vi "HEWH Get Statistics.vi"(4 "Use Emerson 5700?":bool, 6 "Emerson Flow Meter Data Output":T1, 8 "Error In":errorcluster, 10 "Elapsed Time (sec)":dbl, 11 "Core HEWH Data in":T2 {"Test Patten Setup"."PRAT/RLT Sequence"."Time" format="%<%H:%M:%S>t"; "Test Patten Setup"."Total Gallons Schedule" format="%.2f"}) -> (0 "Error Out":errorcluster, 1 "Mean,SD,Var,Max,Min Array":string[][](array[string]), 3 "Draw Stats Out":dbl[][](array[numeric]))   [LabVIEW 2016]
uses:
  Type Definitions/HEWH Output Information.ctl
  Type Definitions/HEWH Draw Pattern Setup.ctl
  Type Definitions/PRAT Test.ctl
  Utility/Save File/File Setup (Public)/Type Definition/Save File HEWH Heating Control Mode.ctl
  Draw Water Specific/Type Definitions/Terminate Draw Conditions.ctl
  Type Definitions/HEWH Start Conditions.ctl
  Draw Water Specific/Type Definitions/Check Special Condtions.ctl
  Draw Water Specific/Type Definitions/HEWH Special Condition Check.ctl
  Type Definitions/HEWH Draw Flag ENUM.ctl
  Type Definitions/HEWH Specific DAQ.ctl
  Type Definitions/HEWH Power Data.ctl
  Type Definitions/HEWH Power Elements.ctl
  Utility/Type Definitions/UTILITY Power Analyzer.ctl
  Type Definitions/HEWH Calc and Calibration.ctl
  Utility/Save File/File Setup (Public)/Type Definition/Save File DOE LabView Program.ctl
  Custom Instrument Control/MW100/Type Definitions/Station ID Selector.ctl
  Drivers/Emerson 5700 Transmitter/Type Definitions/Emerson 5700 Data.ctl
  Utility/Save File/File Setup.lvlib
panel:
  # "Draw Pattern Setup (24 Hour)"
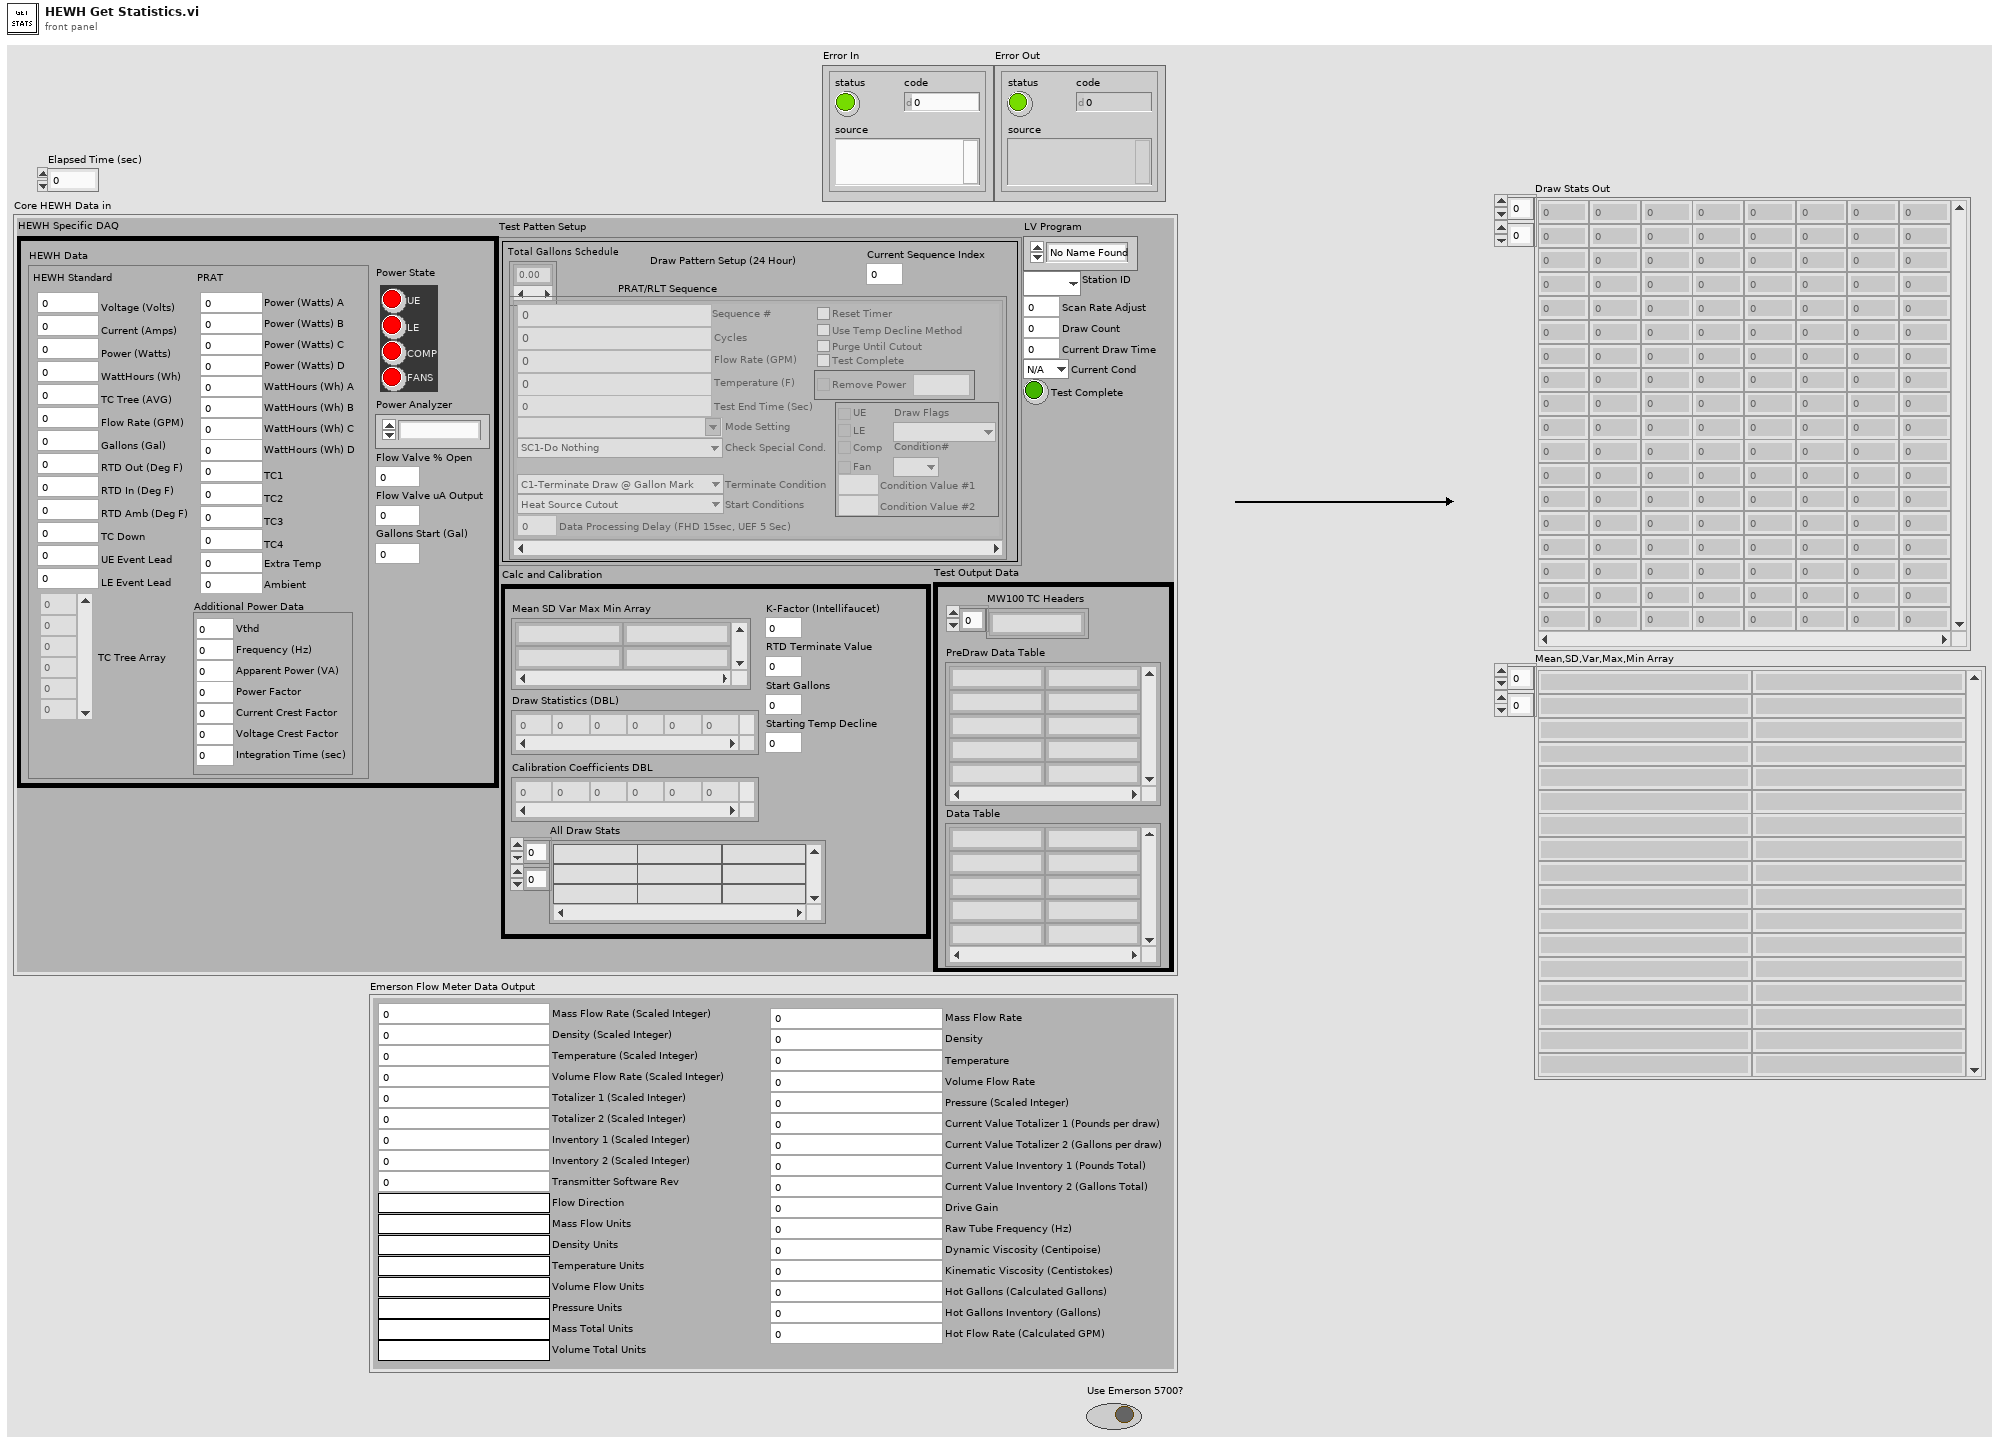
[diagram p1: front panel]
types:
  T1 = typedef "Emerson 5700 Data.ctl" = cluster{"Mass Flow Rate (Scaled Integer)":u16, "Density (Scaled Integer)":u16, "Temperature (Scaled Integer)":u16, "Volume Flow Rate (Scaled Integer)":u16, "Totalizer 1 (Scaled Integer)":u16, "Totalizer 2 (Scaled Integer)":u16, "Transmitter Software Rev":u16, "Flow Direction":string, "Mass Flow Units":string, "Density Units":string, "Temperature Units":string, "Volume Flow Units":string, "Pressure Units":string, "Mass Total Units":string, "Volume Total Units":string, "Inventory 1 (Scaled Integer)":u16, "Inventory 2 (Scaled Integer)":u16, "Mass Flow Rate":dbl, "Density":dbl, "Temperature":dbl, "Volume Flow Rate":dbl, "Pressure (Scaled Integer)":u16, "Current Value Totalizer 1 (Pounds per draw)":dbl, "Current Value Totalizer 2 (Gallons per draw)":dbl, "Current Value Inventory 1 (Pounds Total)":dbl, "Current Value Inventory 2 (Gallons Total)":dbl, "Drive Gain":dbl, "Raw Tube Frequency (Hz)":dbl, "Dynamic Viscosity (Centipoise)":dbl, "Kinematic Viscosity (Centistokes)":dbl, "Hot Gallons (Calculated Gallons)":dbl, "Hot Flow Rate (Calculated GPM)":dbl, "Hot Gallons Inventory (Gallons)":dbl}
  T2 = typedef "HEWH Output Information.ctl" = cluster{"Scan Rate Adjust":dbl, "Draw Count":i32, "Test Patten Setup":T3, "HEWH Specific DAQ":T11, "Test Output Data":cluster{"PreDraw Data Table":string[][], "Data Table":string[][], "MW100 TC Headers":string[]}, "Calc and Calibration":T15, "Current Draw Time":dbl, "LV Program":T16, "Station ID":T17, "Current Cond":T9, "Test Complete":bool}
  T3 = typedef "HEWH Draw Pattern Setup.ctl" = cluster{"Total Gallons Schedule":dbl[], "PRAT/RLT Sequence":T4[], "Current Sequence Index":i32}
  T4 = typedef "PRAT Test.ctl" = cluster{"Sequence #":dbl, "Cycles":i32, "Mode Setting":T5, "Flow Rate (GPM)":dbl, "Temperature (F)":dbl, "Reset Timer":bool, "Use Temp Decline Method":bool, "Terminate Condition":T6, "Condition Value #1":dbl, "UE":bool, "LE":bool, "Comp":bool, "Fan":bool, "Test End Time (Sec)":dbl, "Purge Until Cutout":bool, "Start Conditions":T7, "Condition Value #2":dbl, "Remove Power":bool, "Time":dbl, "Check Special Cond.":T8, "Condition#":T9, "Draw Flags":T10, "Data Processing Delay (FHD 15sec, UEF 5 Sec)":dbl, "Test Complete":bool}
  T5 = typedef "File Setup.lvlib/Save File HEWH Heating Control Mode.ctl" = string
  T6 = typedef "Terminate Draw Conditions.ctl" = enum16{"C1-Terminate Draw @ Gallon Mark", "C2-Special Last Draw (HU Test)", "C3-RTD Out <=", "C4-Mean Tank Temp <=", "C5-Decrease RTD Out (Deg F)", "C6-Time (Seconds)", "C7-Until Any Heat Source", "C8-Specific Heat Source", "C9-Do Nothing"}
  T7 = typedef "HEWH Start Conditions.ctl" = enum16{"Heat Source Cutout", "At Time (Seconds)", "Every X (Seconds)", "T2 >= X° Below Setpoint", "Seconds From Complete", "Wait for LE & Comp Cutout", "Wait for Comp Cutout", "Wait for LE Cutout", "Wait for UE Cutout"}
  T8 = typedef "Check Special Condtions.ctl" = enum16{"SC1-Do Nothing", "SC2-Check Heat Source (On-C2/Off-C1)", "SC3-Check Skip Condition", "SC4-Check Heat Source ON/Fail"}
  T9 = typedef "HEWH Special Condition Check.ctl" = enum16{"N/A", "C1", "C2", "Reset/Fail", "Skip Draw Sequence"}
  T10 = typedef "HEWH Draw Flag ENUM.ctl" = enum16{"N/A", "None(0)", "Sml(1)", "Med(2)", "SmlMed(3)", "Lrg(4)", "SmlLrg(5)", "MedLrg(6)", "SmlMedLrg(7)"}
  T11 = typedef "HEWH Specific DAQ.ctl" = cluster{"HEWH Data":T12, "Flow Valve % Open":dbl, "Power State":T13, "Power Analyzer":T14, "Flow Valve uA Output":i32, "Gallons Start (Gal)":dbl}
  T12 = typedef "HEWH Power Data.ctl" = cluster{"HEWH Standard":cluster{"Voltage (Volts)":dbl, "Current (Amps)":dbl, "Power (Watts)":dbl, "WattHours (Wh)":dbl, "TC Tree (AVG)":dbl, "Flow Rate (GPM)":dbl, "Gallons (Gal)":dbl, "RTD Out (Deg F)":dbl, "RTD In (Deg F)":dbl, "RTD Amb (Deg F)":dbl, "TC Down":dbl, "UE Event Lead":i32, "LE Event Lead":i32, "TC Tree Array":dbl[]}, "PRAT":cluster{"Power (Watts) A":dbl, "Power (Watts) B":dbl, "Power (Watts) C":dbl, "Power (Watts) D":dbl, "TC1":dbl, "TC2":dbl, "TC3":dbl, "TC4":dbl, "WattHours (Wh) A":dbl, "WattHours (Wh) B":dbl, "WattHours (Wh) C":dbl, "WattHours (Wh) D":dbl, "Ambient":dbl, "Extra Temp":dbl}, "Additional Power Data":cluster{"Vthd":dbl, "Frequency (Hz)":dbl, "Apparent Power (VA)":dbl, "Power Factor":dbl, "Current Crest Factor":dbl, "Voltage Crest Factor":dbl, "Integration Time (sec)":dbl}}
  T13 = typedef "HEWH Power Elements.ctl" = cluster{"UE":bool, "LE":bool, "COMP":bool, "FANS":bool}
  T14 = typedef "UTILITY Power Analyzer.ctl" = enum16{"", "APLUS", "WT210", "WT500", "WT300", "OSI", "Debug", "WT230", "WT300_1", "WT300_2"}
  T15 = typedef "HEWH Calc and Calibration.ctl" = cluster{"Mean SD Var Max Min Array":string[][], "Draw Statistics (DBL)":dbl[][], "Calibration Coefficients DBL":dbl[][], "Start Gallons":dbl, "Starting Temp Decline":dbl, "K-Factor (Intellifaucet)":dbl, "All Draw Stats":string[][], "RTD Terminate Value":dbl}
  T16 = typedef "File Setup.lvlib/Save File DOE LabView Program.ctl" = enum16{"No Name Found", "DOE Stand", "Dishwasher Kitchen", "Portable Stand", "HEWH", "Dryer", "Dryer WILT", "HCC", "PRAT", "HEWH RLT", "Refrigeration"}
  T17 = typedef "Station ID Selector.ctl" = enum16{"", "A", "B", "C", "D", "Global"}
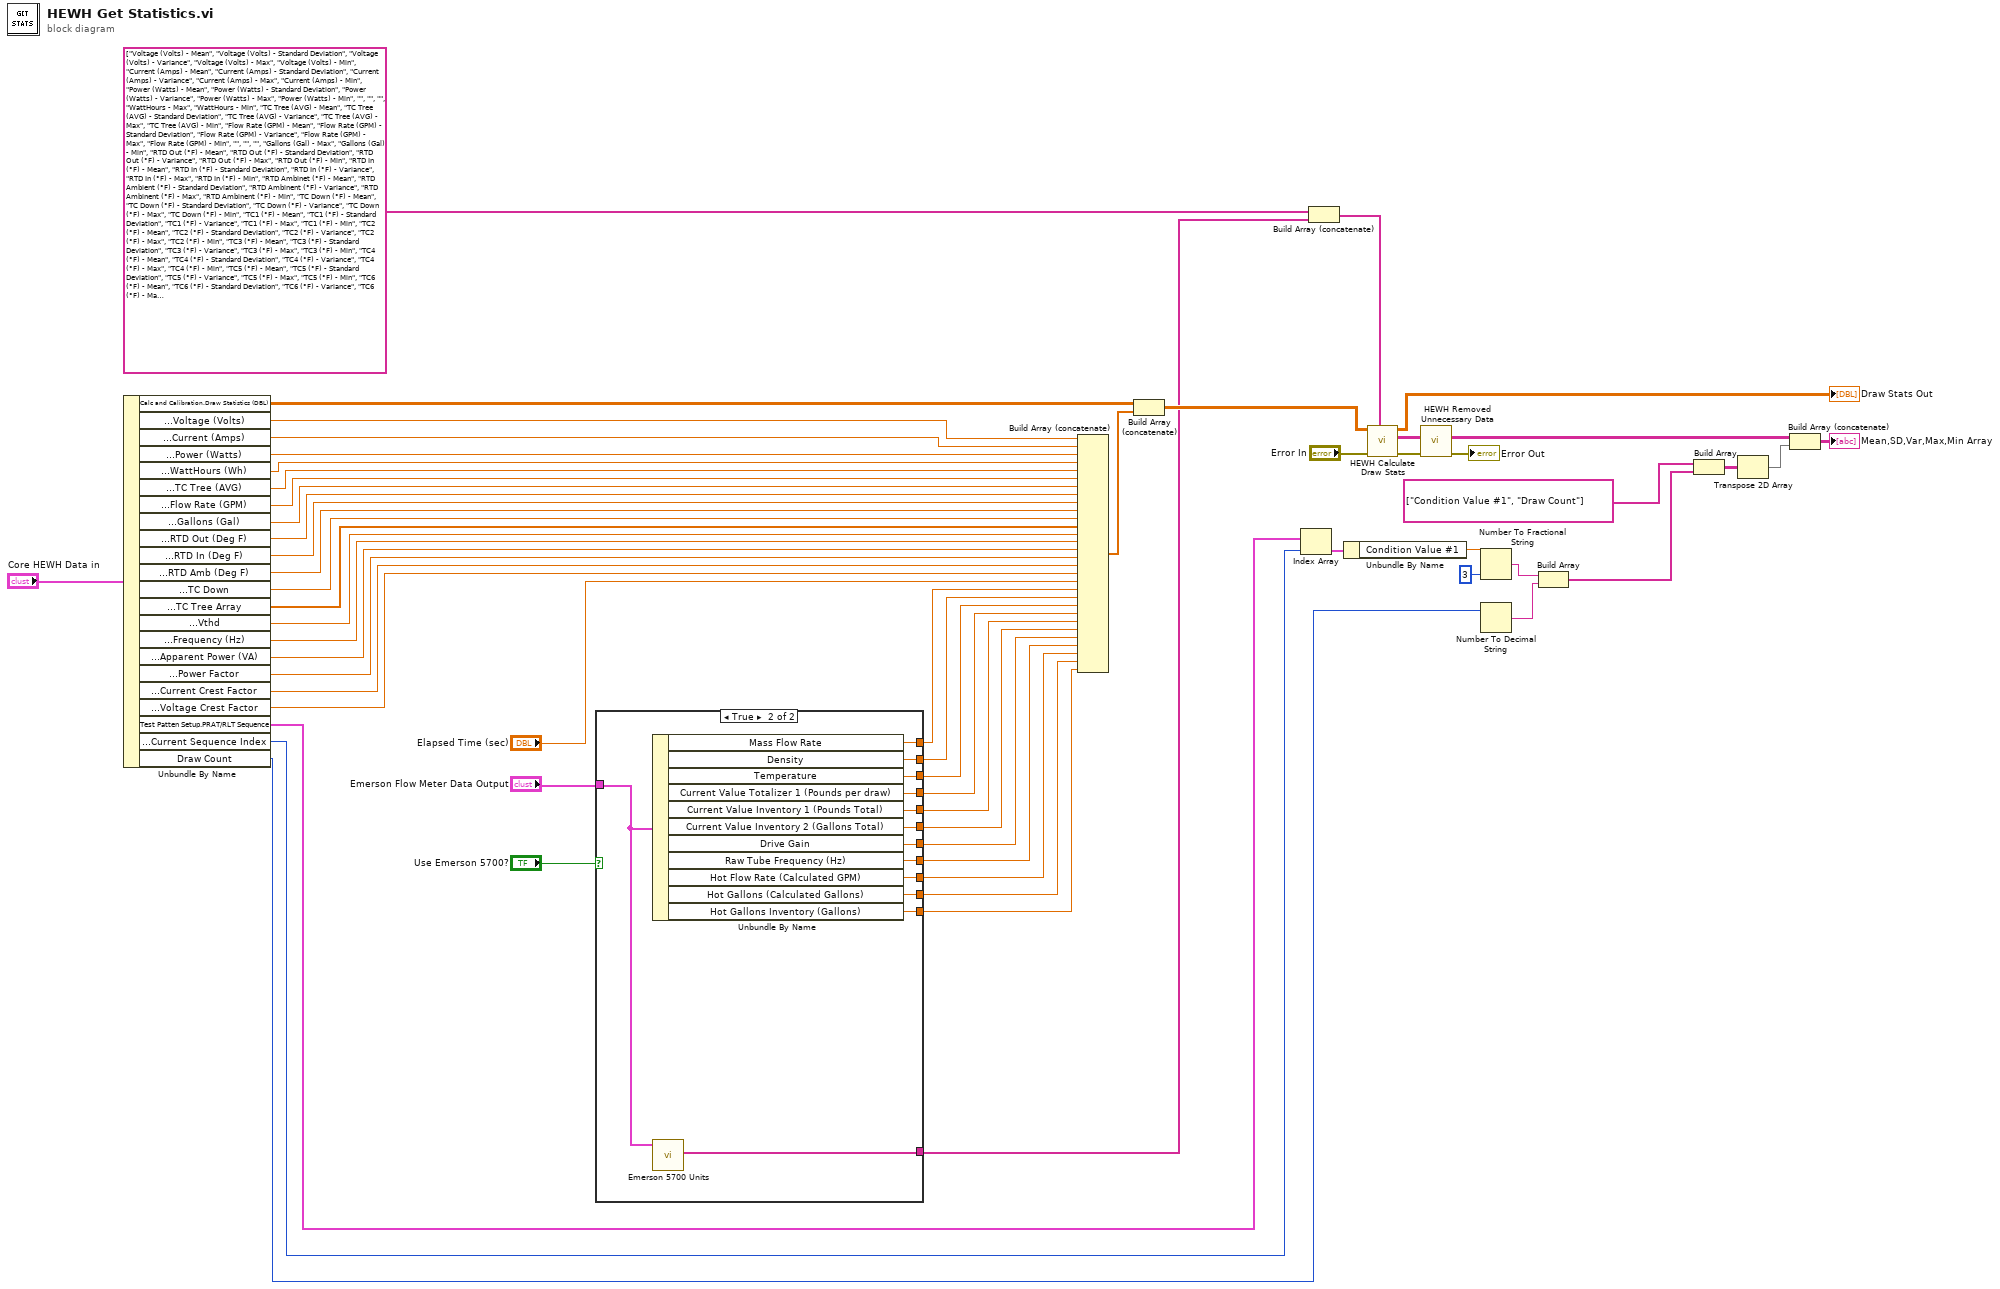
[diagram p0: block diagram]
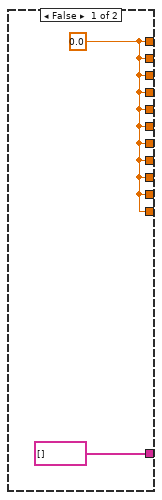
[diagram p2: hidden frame]
diagram:
  n1 = Unbundle By Name("Core HEWH Data in") -> ("Calc and Calibration.Draw Statistics (DBL)"=w49:dbl[][], "HEWH Specific DAQ.HEWH Data.HEWH Standard.Voltage (Volts)"=w30:dbl, "HEWH Specific DAQ.HEWH Data.HEWH Standard.Current (Amps)"=w31:dbl, "HEWH Specific DAQ.HEWH Data.HEWH Standard.Power (Watts)"=w32:dbl, "HEWH Specific DAQ.HEWH Data.HEWH Standard.WattHours (Wh)"=w33:dbl, "HEWH Specific DAQ.HEWH Data.HEWH Standard.TC Tree (AVG)"=w34:dbl, "HEWH Specific DAQ.HEWH Data.HEWH Standard.Flow Rate (GPM)"=w35:dbl, "HEWH Specific DAQ.HEWH Data.HEWH Standard.Gallons (Gal)"=w36:dbl, "HEWH Specific DAQ.HEWH Data.HEWH Standard.RTD Out (Deg F)"=w37:dbl, "HEWH Specific DAQ.HEWH Data.HEWH Standard.RTD In (Deg F)"=w38:dbl, "HEWH Specific DAQ.HEWH Data.HEWH Standard.RTD Amb (Deg F)"=w39:dbl, "HEWH Specific DAQ.HEWH Data.HEWH Standard.TC Down"=w40:dbl, "HEWH Specific DAQ.HEWH Data.HEWH Standard.TC Tree Array"=w41:dbl[], "HEWH Specific DAQ.HEWH Data.Additional Power Data.Vthd"=w42:dbl, "HEWH Specific DAQ.HEWH Data.Additional Power Data.Frequency (Hz)"=w43:dbl, "HEWH Specific DAQ.HEWH Data.Additional Power Data.Apparent Power (VA)"=w44:dbl, "HEWH Specific DAQ.HEWH Data.Additional Power Data.Power Factor"=w45:dbl, "HEWH Specific DAQ.HEWH Data.Additional Power Data.Current Crest Factor"=w46:dbl, "HEWH Specific DAQ.HEWH Data.Additional Power Data.Voltage Crest Factor"=w47:dbl, "Test Patten Setup.PRAT/RLT Sequence"=w51:T4[], "Test Patten Setup.Current Sequence Index"=w52:i32, "Draw Count"=w24:i32)
  n2 = case shown="True" "Use Emerson 5700?" {
    tunnel: "Emerson Flow Meter Data Output" -> [_ w73]
    tunnel: [string[] [] w72] -> w6
    tunnel: [w59 w71] -> w14
    tunnel: [w59 w70] -> w13
    tunnel: [w59 w69] -> w12
    tunnel: [w59 w68] -> w11
    tunnel: [w59 w67] -> w10
    tunnel: [w59 w66] -> w9
    tunnel: [w59 w65] -> w5
    tunnel: [w59 w64] -> w4
    tunnel: [w59 w63] -> w3
    tunnel: [w59 w62] -> w2
    tunnel: [w59 w61] -> w1
    frame False {
      w59 = 0.0 ("Mass Flow Rate")
    }
    frame True {
      n3 = Unbundle By Name(w73) -> ("Mass Flow Rate"=w71:dbl, "Density"=w70:dbl, "Temperature"=w69:dbl, "Current Value Totalizer 1 (Pounds per draw)"=w68:dbl, "Current Value Inventory 1 (Pounds Total)"=w67:dbl, "Current Value Inventory 2 (Gallons Total)"=w66:dbl, "Drive Gain"=w65:dbl, "Raw Tube Frequency (Hz)"=w64:dbl, "Hot Flow Rate (Calculated GPM)"=w63:dbl, "Hot Gallons (Calculated Gallons)"=w62:dbl, "Hot Gallons Inventory (Gallons)"=w61:dbl)
      n4 = call "Emerson 5700 Units.vi"("Emerson Flow Meter Data Input"=w73) -> ("Units with Mean, STD, ect"=w72:string[])  [unwired: 7 in, 3 out]
    }
  }
  n5 = Build Array (concatenate)(w30, w31, w32, w33, w34, w35, w36, w37, w38, w39, w40, w41, w42, w43, w44, w45, w46, w47, "Elapsed Time (sec)", w14, w13, w12, w11, w10, w9, w5, w4, w3, w2, w1) -> (w48:dbl[])
  n6 = Build Array (concatenate)(w49, w48) -> (w58:dbl[][])
  n7 = Index Array(array=w51, index=w52) -> (element=w50:T4)
  n8 = Build Array (concatenate)(string[] ["Voltage (Volts) - Mean", "Voltage (Volts) - Standard Deviation", "Voltage (Volts) - Variance", "Voltage (Volts) - Max", "Voltage (Volts) - Min", "Current (Amps) - Mean", "Current (Amps) - Standard Deviation", "Current (Amps) - Variance", "Current (Amps) - Max", "Current (Amps) - Min", "Power (Watts) - Mean", "Power (Watts) - Standard Deviation", "Power (Watts) - Variance", "Power (Watts) - Max", "Power (Watts) - Min", "", "", "", "WattHours - Max", "WattHours - Min", "TC Tree (AVG) - Mean", "TC Tree (AVG) - Standard Deviation", "TC Tree (AVG) - Variance", "TC Tree (AVG) - Max", "TC Tree (AVG) - Min", "Flow Rate (GPM) - Mean", "Flow Rate (GPM) - Standard Deviation", "Flow Rate (GPM) - Variance", "Flow Rate (GPM) - Max", "Flow Rate (GPM) - Min", "", "", "", "Gallons (Gal) - Max", "Gallons (Gal) - Min", "RTD Out (°F) - Mean", "RTD Out (°F) - Standard Deviation", "RTD Out (°F) - Variance", "RTD Out (°F) - Max", "RTD Out (°F) - Min", "RTD In (°F) - Mean", "RTD In (°F) - Standard Deviation", "RTD In (°F) - Variance", "RTD In (°F) - Max", "RTD In (°F) - Min", "RTD Ambinet (°F) - Mean", "RTD Ambient (°F) - Standard Deviation", "RTD Ambinent (°F) - Variance", "RTD Ambinent (°F) - Max", "RTD Ambinent (°F) - Min", "TC Down (°F) - Mean", "TC Down (°F) - Standard Deviation", "TC Down (°F) - Variance", "TC Down (°F) - Max", "TC Down (°F) - Min", "TC1 (°F) - Mean", "TC1 (°F) - Standard Deviation", "TC1 (°F) - Variance", "TC1 (°F) - Max", "TC1 (°F) - Min", "TC2 (°F) - Mean", "TC2 (°F) - Standard Deviation", "TC2 (°F) - Variance", "TC2 (°F) - Max", "TC2 (°F) - Min", "TC3 (°F) - Mean", "TC3 (°F) - Standard Deviation", "TC3 (°F) - Variance", "TC3 (°F) - Max", "TC3 (°F) - Min", "TC4 (°F) - Mean", "TC4 (°F) - Standard Deviation", "TC4 (°F) - Variance", "TC4 (°F) - Max", "TC4 (°F) - Min", "TC5 (°F) - Mean", "TC5 (°F) - Standard Deviation", "TC5 (°F) - Variance", "TC5 (°F) - Max", "TC5 (°F) - Min", "TC6 (°F) - Mean", "TC6 (°F) - Standard Deviation", "TC6 (°F) - Variance", "TC6 (°F) - Max", "TC6 (°F) - Min", "", "", "", "Total Harmonic Distortion (%V) - Max", "Total Harmonic Distortion (%V) - Min", "Frequency (Hz) - Mean ", "Frequency (Hz) - Standard Deviation", "Frequency (Hz) - Variance", "Frequency (Hz) - Max", "Frequency (Hz) - Min", "Apparent Power (VA) - Mean", "Apparent Power (VA) - Standard Deviation", "Apparent Power (VA) - Variance", "Apparent Power (VA) - Max", "Apparent Power (VA) - Min", "", "", "", "Power Factor - Max", "Power Factor - Min", "", "", "", "Current Crest Factor - Max", "Current Crest Factor - Min", "", "", "", "Voltage Crest Factor - Max", "Voltage Crest Factor - Min", "", "", "", "Elapsed Time (Sec) - Max", "Elapsed Time (Sec) - Min"], w6) -> (w7:string[])
  n9 = Unbundle By Name(w50) -> ("Condition Value #1"=w26:dbl)
  n10 = call "HEWH Calculate Draw Stats.vi"("Headers"=w7, "Error In"="Error In", "Draw Stats"=w58) -> ("Error Out"=w57:errorcluster, "Data With Headers"=w54:string[][], "Draw Stats Out"=→"Draw Stats Out":dbl[][])  [unwired: 6 in]
  n11 = call "HEWH Removed Unnecessary Data.vi"("Error In"=w57, "Data With Headers"=w54) -> ("Error Out"=→"Error Out":errorcluster, "Stat Data Output"=w21:string[][])  [unwired: 7 in, 1 out]
  n12 = Number To Fractional String(number=w26, precision (6)=i16 3) -> (F-format string=w25:string)  [unwired: 2 in]
  n13 = Number To Decimal String(number=w24) -> (decimal integer string=w23:string)  [unwired: 1 in]
  n14 = Build Array(w25, w23) -> (w22:string[])
  n15 = Build Array(string[] ["Condition Value #1", "Draw Count"], w22) -> (w19:string[][])
  n16 = Transpose 2D Array(2D array=w19) -> (transposed array=w18:string[][])
  n17 = Build Array (concatenate)(w21, w18) -> (→"Mean,SD,Var,Max,Min Array":string[][])
